vi "Test MQTT-4.7.3-4.vi"(8 "error in (no error)":errorcluster) -> (0 "error out":errorcluster)   [LabVIEW 2013]
uses:
  <vilib>/addons/_JKI Toolkits/Caraya/classes/Test/Test.lvclass
  <vilib>/addons/_JKI Toolkits/Caraya/classes/Assert/Assert.lvclass
  source/TopicFilter/TopicFilter.lvclass
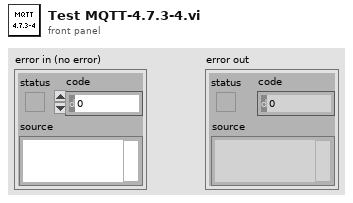
[diagram p1: front panel]
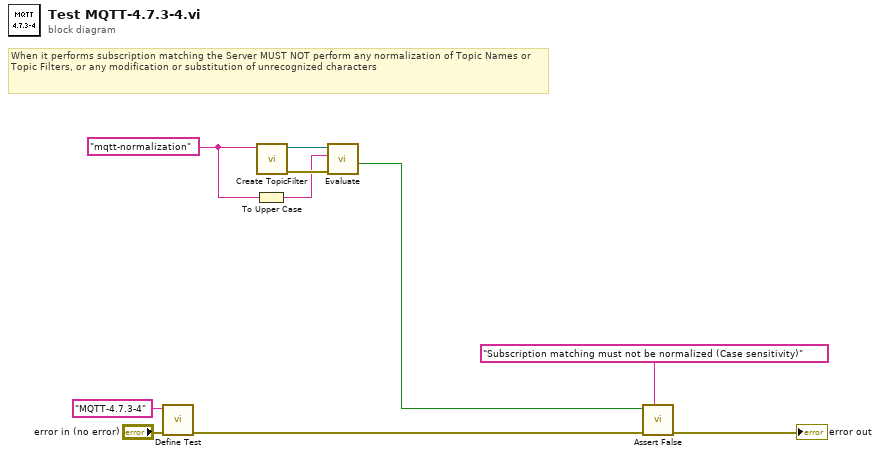
[diagram p0: block diagram]
diagram:
  w2 = "mqtt-normalization" ("Label (VI Title)")
  # "When it performs subscription matching the Server MUST NOT perform any normalization of Topic Names or Topic Filters, or any modification or substitution of unrecognized characters"
  n1 = call <vilib>:"Define Test.vi"("error in (no error)"="error in (no error)", "Label (VI Title)"="MQTT-4.7.3-4") -> ("error out"=w7:errorcluster)  [unwired: 9 in]
  n2 = To Upper Case(1:w2) -> (0:w3:string)
  n3 = call "Create TopicFilter.vi"("Topic Filter"=w2) -> ("error out"=w4:errorcluster, "TopicFilter out"=w5:refnum<class "TopicFilter.lvclass">)  [unwired: 9 in]
  n4 = call "Evaluate.vi"("error in (no error)"=w4, "Topic"=w3, "TopicFilter in"=w5) -> ("Match"=w1:bool)  [unwired: 5 in, 3 out]
  n5 = call <vilib>:"Assert False.vi"("Label"="Subscription matching must not be normalized (Case sensitivity)", "error in (no error)"=w7, "False?"=w1) -> ("error out"=→"error out":errorcluster)  [unwired: 8 in]
